vi "SQL Execute.vi"(8 "error in (no error)":errorcluster, 10 "Command Text":string, 11 "SQLite_API in":refnum<class "SQLite_API.lvclass">) -> (0 "error out":errorcluster, 1 "FirstRow":string[](array[string]), 2 "Datas":string[][](table), 3 "SQLite_API out":refnum<class "SQLite_API.lvclass">, 4 "Rows Fetched":i32)   [LabVIEW 2021, in "SQLite_API.lvclass"]
uses:
  <userlib>/John_Lib/DataBase/SQLite_API/SQLite_API.lvclass
  <userlib>/John_Lib/DataBase/SQLite_API/SQLite_API.lvclass/SQLite_API.ctl
  <vilib>/drjdpowell/SQLite Library/SQL Connection/Connection.lvclass
  <vilib>/drjdpowell/SQLite Library/SQLite.lvlib
  <vilib>/drjdpowell/SQLite Library/SQL Connection/Execute SQL (No results).vi
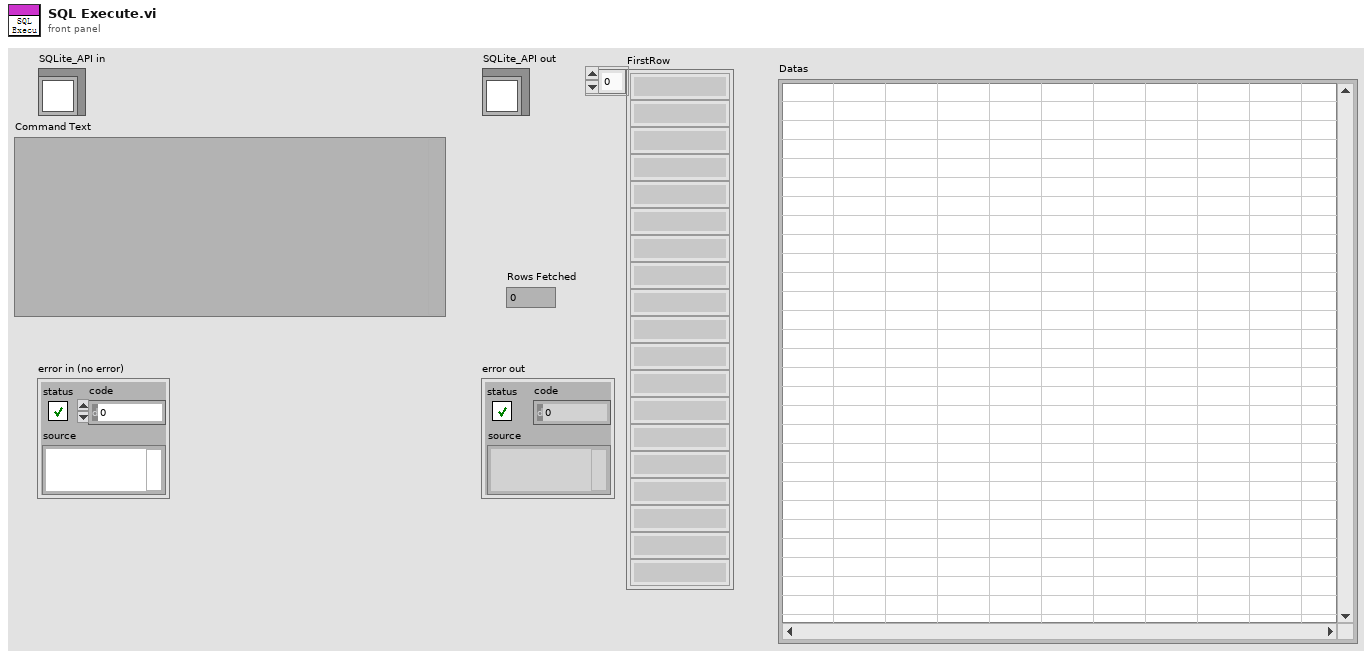
[diagram p1: front panel]
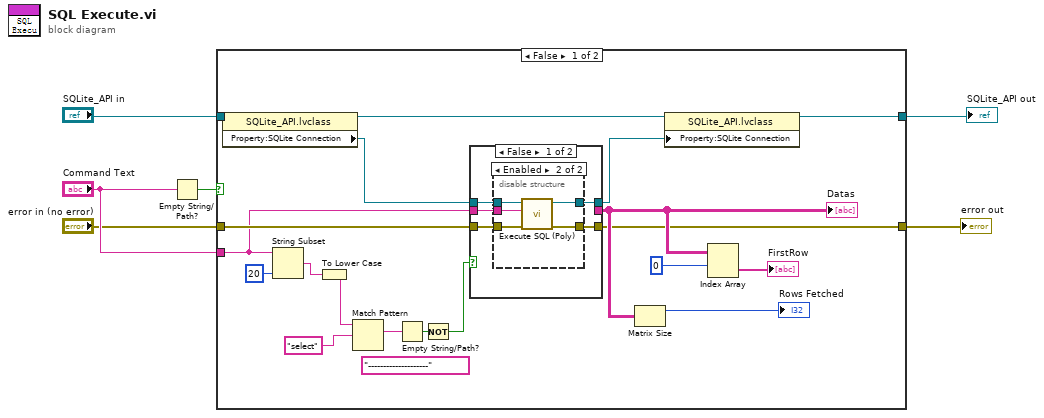
[diagram p0: block diagram]
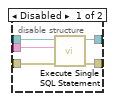
[diagram p2: hidden frame]
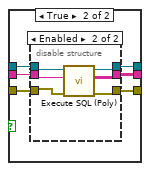
[diagram p3: hidden frame]
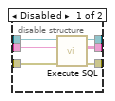
[diagram p4: hidden frame]
diagram:
  n1 = Empty String/Path?(string/path="Command Text") -> (empty?=w6:bool)
  n2 = case shown="False" w6 {
    tunnel: [w13 w60] -> w5
    tunnel: "SQLite_API in" -> [w25 w60]
    tunnel: "Command Text" -> [w14 _]
    tunnel: "error in (no error)" -> [w15 w59]
    tunnel: [w7 w59] -> w1
    frame False {
      (unwired) "--------------------" ("string")
      n3 = property class="SQLite_API.lvclass"(reference=w25) -> (reference out=w24:refnum<class "SQLite_API.lvclass">, "Property:SQLite Connection"=w17:refnum<class "Connection.lvclass">)  [unwired: 1 in, 1 out]
      n4 = String Subset(string=w14, length (rest)=20 ("length (rest)")) -> (substring=w22:string)  [unwired: 1 in]
      n5 = To Lower Case(string=w22) -> (all lower case string=w23:string)
      n6 = Match Pattern(string=w23, regular expression="select") -> (match substring=w19:string)  [unwired: 1 in, 3 out]
      n7 = Empty String/Path?(string/path=w19) -> (empty?=w18:bool)
      n8 = Not(x=w18) -> (.not. x?=w16:bool)
      n9 = case shown="False" w16 {
        tunnel: w17 -> [w30 w46]
        tunnel: [_ w45] -> w9
        tunnel: [w29 w44] -> w12
        tunnel: w15 -> [w27 w43]
        tunnel: [w26 w42] -> w7
        tunnel: w14 -> [w28 w41]
        frame False {
          n10 = disable-structure shown="Enabled" {
            disable-tunnel: w30 -> [w35 w40]
            disable-tunnel: [w34 w38] -> w29
            disable-tunnel: w28 -> [w33 w39]
            disable-tunnel: w27 -> [w32 w37]
            disable-tunnel: [w31 w36] -> w26
            frame Disabled {
              n11 = call <vilib>:"Execute Single SQL Statement.vi"("error in (no error)"=w32, "SQL statement"=w33, "SQLite Connection in"=w35) -> ("error out"=w31:errorcluster, "SQLite Connection"=w34:refnum<class "Connection.lvclass">)  [unwired: 7 in]
            }
            frame Enabled {
              n12 = call-poly <vilib>:"Execute SQL (Poly).vi"("error in (no error)"=w37, "SQL"=w39, "SQLite Connection in"=w40) -> ("error out"=w36:errorcluster, "SQLite Connection"=w38:refnum<class "Connection.lvclass">)  [unwired: 7 in]
            }
          }
        }
        frame True {
          n13 = disable-structure shown="Enabled" {
            disable-tunnel: w46 -> [w52 w58]
            disable-tunnel: [w51 w53] -> w45
            disable-tunnel: [w50 w57] -> w44
            disable-tunnel: w43 -> [w49 w56]
            disable-tunnel: [w48 w54] -> w42
            disable-tunnel: w41 -> [w47 w55]
            frame Disabled {
              n14 = call <vilib>:"Execute SQL.vi"("error in (no error)"=w49, "SQL"=w47, "SQLite Connection in"=w52) -> ("error out"=w48:errorcluster, "Result Set"=w51:string[][], "SQLite Connection"=w50:refnum<class "Connection.lvclass">)  [unwired: 5 in, 1 out]
            }
            frame Enabled {
              n15 = call-poly <vilib>:"Execute SQL (Poly).vi"("error in (no error)"=w56, "SQL"=w55, "SQLite Connection in"=w58) -> ("error out"=w54:errorcluster, "Result Set"=w53:string[][], "SQLite Connection"=w57:refnum<class "Connection.lvclass">)  [unwired: 5 in, 1 out]
            }
          }
        }
      }
      "Datas" <- w9
      n16 = Matrix Size(0:w9) -> (1:→"Rows Fetched":i32)  [unwired: 1 out]
      n17 = property class="SQLite_API.lvclass"(reference=w24, "Property:SQLite Connection"=w12) -> (reference out=w13:refnum<class "SQLite_API.lvclass">)  [unwired: 1 in, 1 out]
      n18 = Index Array(array=w9, index (row)=0) -> (element=→"FirstRow":string[])  [unwired: 1 in]
    }
    frame True {
    }
  }
  "error out" <- w1
  "SQLite_API out" <- w5
